vi "Custom User Scripting For New Simple Accessor VI.vi"(8 "error in":errorcluster, 10 "Write VI":refnum<vi>, 11 "Read VI":refnum<vi>) -> (0 "error out":errorcluster)   [LabVIEW 2019]
doc: "When \"New >> VI For Data Member Access...\" is used to create VIs, this subVI will be invoked if the VIs are created successfully after all other work to create the VIs has been completed. Users may edit this subVI to add any instructions they wish for customizations of the newly generated VIs."
uses:
  <vilib>/Utility/traverseref.llb/TRef TravTarget.ctl
  <vilib>/Utility/traverseref.llb/VI Scripting - Traverse.lvlib
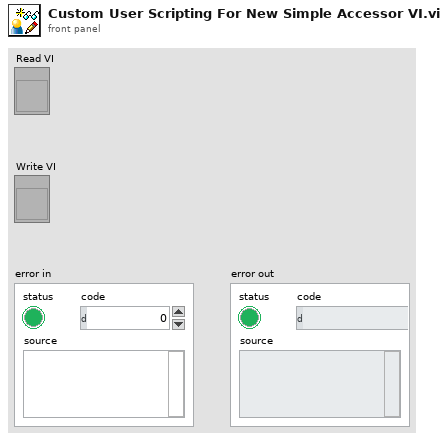
[diagram p1: front panel]
types:
  T1 = typedef "TRef TravTarget.ctl" = enum16{"FP", "BD", "Other"}
  T2 = typedef "LVRectTypeDef.ctl" = cluster{"Left":i16, "Top":i16, "Right":i16, "Bottom":i16}
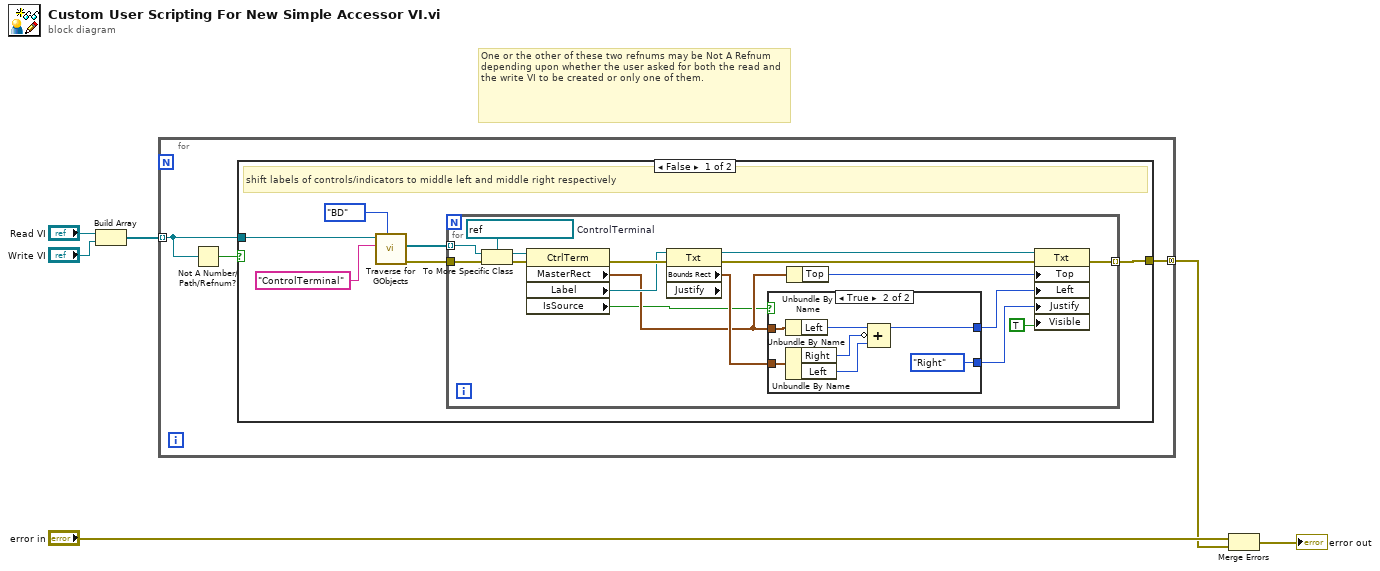
[diagram p0: block diagram]
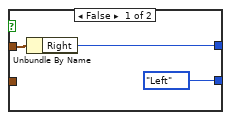
[diagram p2: hidden frame]
diagram:
  # "One or the other of these two refnums may be Not A Refnum depending upon whether the user asked for both the read and the write VI to be created or only one of them."
  n1 = Build Array("Read VI", "Write VI") -> (w3:refnum<vi>[])
  n2 = for {
    tunnel: w3 -> [w8] mode=indexing
    tunnel: [w7] -> w1 mode=concatenating
    n3 = Not A Number/Path/Refnum?(number/path/refnum=w8) -> (NaN/Path/Refnum?=w9:bool)
    n4 = case shown="False" w9 {
      tunnel: w8 -> [w11 _]
      tunnel: [w10 _] -> w7
      frame False {
        # "shift labels of controls/indicators to middle left and middle right respectively"
        n5 = call <vilib>:"Traverse for GObjects.vi"("Traverse Target"=TRef_TravTarget."BD", "Class Name"="ControlTerminal", "VI Refnum"=w11) -> ("error out"=w14:errorcluster, "References"=w13:refnum<vi>[])  [unwired: 5 in, 2 out]
        n6 = for {
          tunnel: w13 -> [w23] mode=indexing
          tunnel: w14 -> [w31]
          tunnel: [w32] -> w10 mode=indexing
          w22 = refnum<vi> refnum  # ControlTerminal
          n7 = To More Specific Class(target class=w22, reference=w23, error in=w31) -> (specific class reference=w20:refnum<vi>, error out=w21:errorcluster)
          n8 = property class="CtrlTerm"(reference=w20, error in=w21) -> (error out=w19:errorcluster, "MasterRect"=w17:T2, "Label"=w18:refnum<vi>, "IsSource"=w16:bool)  [unwired: 1 out]
          n9 = property class="Txt" props=["Bounds Rect", "Justify"](reference=w18, error in=w19) -> (reference out=w30:refnum<vi>, error out=w28:errorcluster, "Bounds Rect"=w27:T2)  [unwired: 1 out]
          n10 = case shown="True" w16 {
            tunnel: w17 -> [w35 w42]
            tunnel: w27 -> [_ w40]
            tunnel: [w34 w37] -> w26
            tunnel: [enum16{"Left", "Center", "Right"}."Left" ("Justification") enum16{"Left", "Center", "Right"}."Right" ("Justification")] -> w25
            frame False {
              n11 = Unbundle By Name(w35) -> ("Right"=w34:i16)
            }
            frame True {
              n12 = Unbundle By Name(w42) -> ("Left"=w41:i16)
              n13 = Unbundle By Name(w40) -> ("Right"=w39:i16, "Left"=w38:i16)
              n14 = Compound Arithmetic op=ADD(w41, invert w39, w38) -> (w37:i16)
            }
          }
          n15 = Unbundle By Name(w17) -> ("Top"=w29:i16)
          n16 = property class="Txt"(reference=w30, error in=w28, "Top"=w29, "Left"=w26, "Justify"=w25, "Visible"=TRUE) -> (error out=w32:errorcluster)  [unwired: 1 out]
        }
      }
      frame True {
        # "not a valid ref, so ignore"
      }
    }
  }
  n17 = Merge Errors("error in", w1) -> (→"error out":errorcluster)
